vi "Set_Parameter_Instrument (Json).vi"(8 "error in (no error)":errorcluster caption="entrée d'erreur (pas d'erreur)", 10 "Parameter (Json)":string, 11 "Flash_Jlink en entrée":refnum<class "Flash_P2056.lvclass">) -> (0 "error out":errorcluster caption="sortie d'erreur", 3 "Flash_Jlink en sortie":refnum<class "Flash_P2056.lvclass">)   [LabVIEW 2020, in "Library Test.lvlib" / "Flash_P2056.lvclass"]
uses:
  Flash_P2056.lvclass
  C:/Users/ngarcin/OneDrive - Altyor/Standard TB/Class/Test/Test (Default)/Test (Default).lvclass
  Commun VI/TypeDef/Commande Test/Commande Parameter Flash_P2056.ctl
  Flash_P2056.lvclass/Flash_P2056.ctl
  JSON API/JSON Value/Set from JSON string.vi
  Test_Without_Instr/Test_Without_Inst.lvclass
  JSON API/JSON Value/JSON Value.lvclass
  JSON API/Variant JSON/Variant JSON.lvlib
  JSON API/Get Polymorphic/JSON GetSet.lvlib
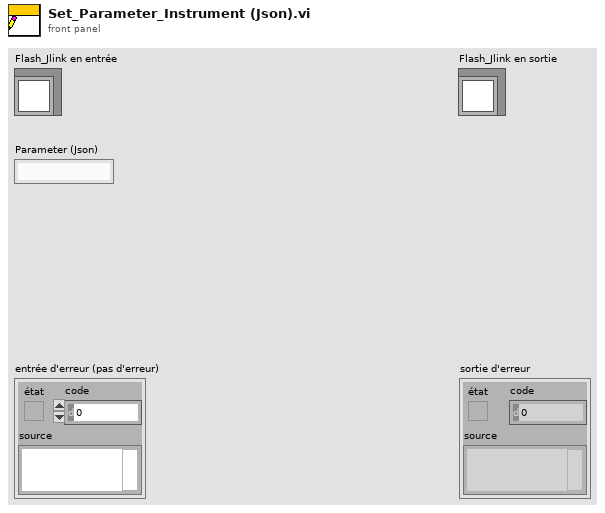
[diagram p1: front panel]
types:
  T1 = typedef "Commande Parameter Flash_P2056.ctl" = cluster{"Path FW":path}
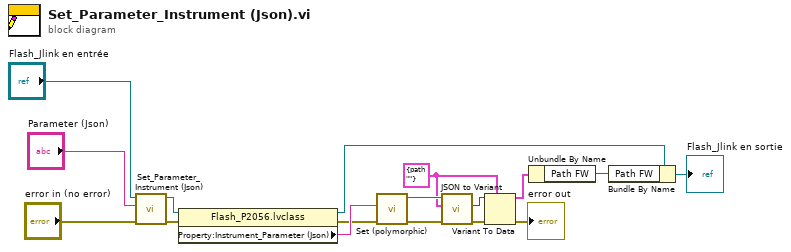
[diagram p0: block diagram]
diagram:
  w2 = T1 {"Path FW"=path ""} ("Cluster")
  n1 = call-parent "Set_Parameter_Instrument (Json).vi"("error in (no error)"="error in (no error)", "Parameter (Json)"="Parameter (Json)", "Test (Default) en entrée"="Flash_Jlink en entrée") -> ("error out"=w7:errorcluster, "Test (Default) en sortie"=w9:refnum<class "Flash_P2056.lvclass">)  [unwired: 7 in]
  n2 = property class="Flash_P2056.lvclass"(reference=w9, error in=w7) -> (reference out=w6:refnum<class "Flash_P2056.lvclass">, error out=w4:errorcluster, "Property:Instrument_Parameter (Json)"=w8:string)
  n3 = call-poly "Set (polymorphic).vi"("error in (no error)"=w4, "JSON stream"=w8) -> ("error out"=w11:errorcluster, "JSON Value out"=w13:refnum<class "JSON Value.lvclass">)  [unwired: 7 in, 1 out]
  n4 = call "JSON to Variant.vi"("error in (no error)"=w11, "Variant (Data Type)"=w2, "JSON Value"=w13) -> ("error out"=w12:errorcluster, "Variant out"=w10:variant)  [unwired: 7 in]
  n5 = Variant To Data(error in=w12, type=w2, Variant=w10) -> (data=w5:T1, error out=→"error out":errorcluster)
  n6 = Unbundle By Name(w5) -> ("Path FW"=w1:path)
  n7 = Bundle By Name(cluster=w6, "Path FW"=w1) -> (→"Flash_Jlink en sortie":refnum<class "Flash_P2056.lvclass">)
